vi "cms50h link.vi"() -> ()   [LabVIEW 2020]
uses:
  <vilib>/Instr/_visa.llb/VISA Configure Serial Port (Instr).vi
panel:
  out "Pulse":bool
  out "PI":ext
  out "SPO2":u8
  out "HR":u8
  out "Bar graph":dbl(slide) scale=0.0..100.0
  out "Waveform Chart 2":dbl(graph)
  out "HEX":u8[](array[numeric]) format="%x"
  out "ASCII":u8[](array[numeric])
  out "read buffer":string
  in  "stop":bool
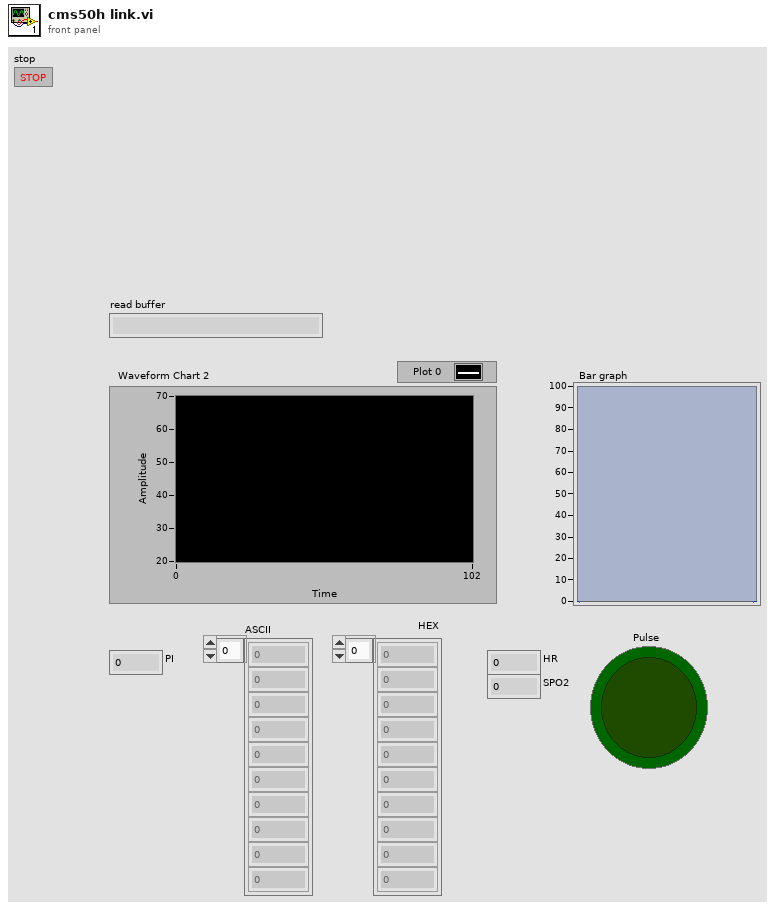
[diagram p1: front panel]
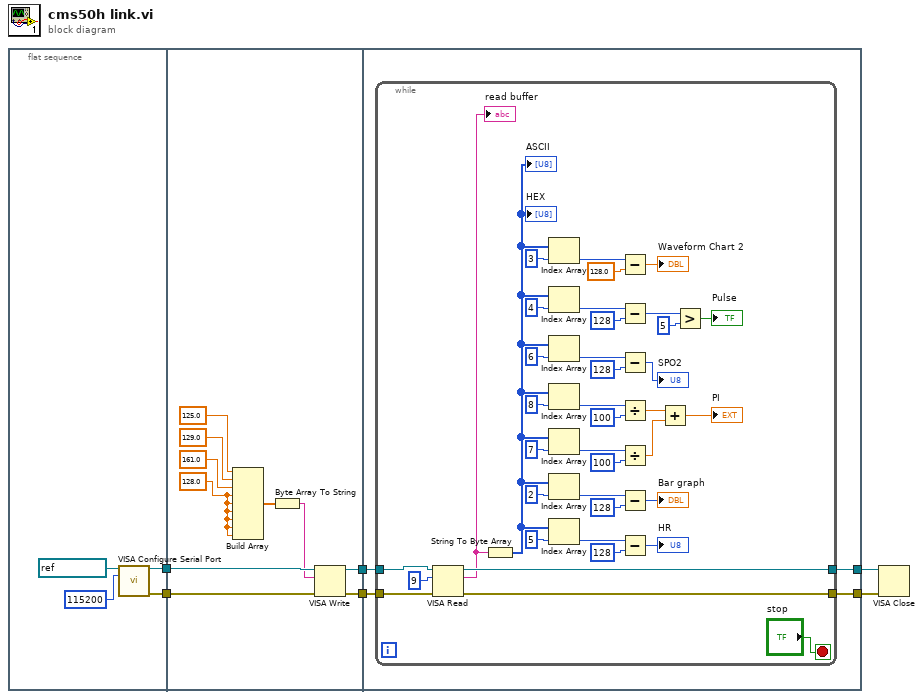
[diagram p0: block diagram]
diagram:
  n1 = flat-sequence {
    tunnel: [w8] -> w6
    tunnel: [w7] -> w5
    tunnel: w6 -> [w15]
    tunnel: w5 -> [w16]
    tunnel: [w14] -> w2
    tunnel: [w13] -> w1
    tunnel: [w22] -> w4
    tunnel: [w21] -> w3
    tunnel: w2 -> [w23]
    tunnel: w1 -> [w24]
    frame #0 {
      n2 = call-poly "VISA Configure Serial Port"("VISA resource name"=refnum<visa-resource-name> "COM11", "baud rate (9600)"=u32 115200) -> ("VISA resource name out"=w7:refnum<visa-resource-name>, "error out"=w8:errorcluster)  [unwired: 12 in]
    }
    frame #1 {
      w17 = 128.0 ("element")
      n3 = Build Array(125.0 ("element"), 129.0 ("element"), 161.0 ("element"), w17, w17, w17, w17, w17, w17) -> (w11:dbl[])
      n4 = Byte Array To String(unsigned byte array=w11) -> (string=w12:string)
      n5 = VISA Write(VISA resource name=w16, write buffer=w12, error in (no error)=w15) -> (VISA resource name out=w14:refnum<visa-resource-name>, error out=w13:errorcluster)  [unwired: 1 out]
    }
    frame #2 {
      n6 = while {
        tunnel: w24 -> [w59]
        tunnel: w23 -> [w60]
        tunnel: [w62] -> w22
        tunnel: [w61] -> w21
        stop <- "stop" stop-if-true
        n7 = VISA Read(VISA resource name=w60, byte count=u32 9, error in (no error)=w59) -> (VISA resource name out=w62:refnum<visa-resource-name>, read buffer=w57:string, error out=w61:errorcluster)  [unwired: 1 out]
        "read buffer" <- w57
        n8 = String To Byte Array(string=w57) -> (unsigned byte array=w31:u8[])
        "ASCII" <- w31
        "HEX" <- w31
        n9 = Index Array(array=w31, index=3) -> (element=w43:u8)
        n10 = Index Array(array=w31, index=4) -> (element=w29:u8)
        n11 = Index Array(array=w31, index=6) -> (element=w48:u8)
        n12 = Index Array(array=w31, index=8) -> (element=w37:u8)
        n13 = Index Array(array=w31, index=7) -> (element=w35:u8)
        n14 = Index Array(array=w31, index=2) -> (element=w44:u8)
        n15 = Index Array(array=w31, index=5) -> (element=w45:u8)
        n16 = Subtract(x=w43, y=128.0 ("x")) -> (x-y=→"Waveform Chart 2":dbl)
        n17 = Subtract(x=w29, y=u8 128) -> (x-y=w27:u8)
        n18 = Subtract(x=w48, y=u8 128) -> (x-y=→"SPO2":u8)
        n19 = Divide(x=w37, y=u8 100) -> (x/y=w33:ext)
        n20 = Divide(x=w35, y=u8 100) -> (x/y=w34:ext)
        n21 = Subtract(x=w44, y=u8 128) -> (x-y=→"Bar graph":u8)
        n22 = Subtract(x=w45, y=u8 128) -> (x-y=→"HR":u8)
        n23 = Add(x=w33, y=w34) -> (x+y=→"PI":ext)
        n24 = Greater?(x=w27, y=u8 5) -> (0:→"Pulse":bool)
      }
    }
  }
  n25 = VISA Close(VISA resource name=w4, error in (no error)=w3) -> ()  [unwired: 1 out]
